vi "Convert Binary to Genealogy.vi"(8 "error in (no error)":errorcluster, 9 "week and serial Bin In":i32=2200123 format="%b", 10 "Vendor Bin In":u8[](array[numeric])=[81, 77, 67] format="%b", 11 "PN Bin In":u8[](array[numeric])=[49, 48, 48, 48, 48, 48, 48, 49] format="%b") -> (0 "error out":errorcluster, 2 "SN out":string="0", 3 "PN out":string="-")   [LabVIEW 2021, in "CAN wrapper.lvlib"]
uses:
  CAN wrapper.lvlib
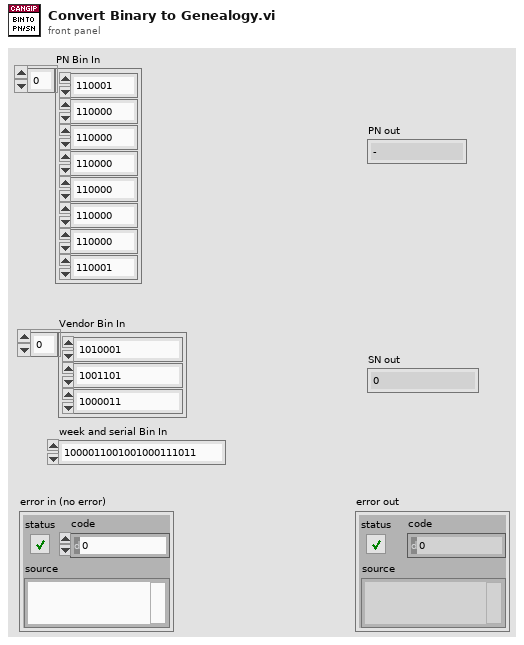
[diagram p1: front panel]
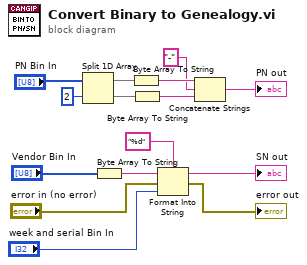
[diagram p0: block diagram]
diagram:
  n1 = Split 1D Array(array="PN Bin In", index=2) -> (first subarray=w7:u8[], second subarray=w6:u8[])
  n2 = Byte Array To String(unsigned byte array="Vendor Bin In") -> (string=w14:string)
  n3 = Byte Array To String(unsigned byte array=w7) -> (string=w5:string)
  n4 = Byte Array To String(unsigned byte array=w6) -> (string=w4:string)
  n5 = Format Into String(format string="%d", initial string=w14, error in="error in (no error)", "week and serial Bin In") -> (resulting string=→"SN out":string, error out=→"error out":errorcluster)
  n6 = Concatenate Strings(w5, "-" ("string"), w4) -> (→"PN out":string)
